vi "SaveModelFile.vi"(8 "error in":errorcluster, 11 "ItemNames":string[][](array[string])) -> (0 "error out":errorcluster)   [LabVIEW 2013]
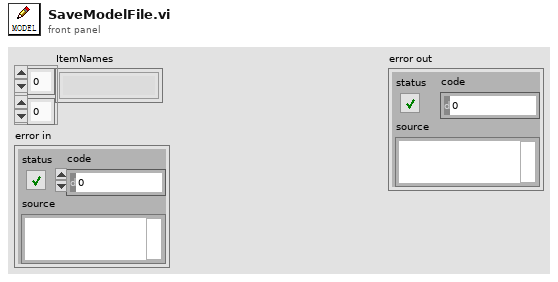
[diagram p1: front panel]
types:
  T1 = enum16{"open", "replace", "create", "open or create", "replace or create", "replace or create with confirmation"}
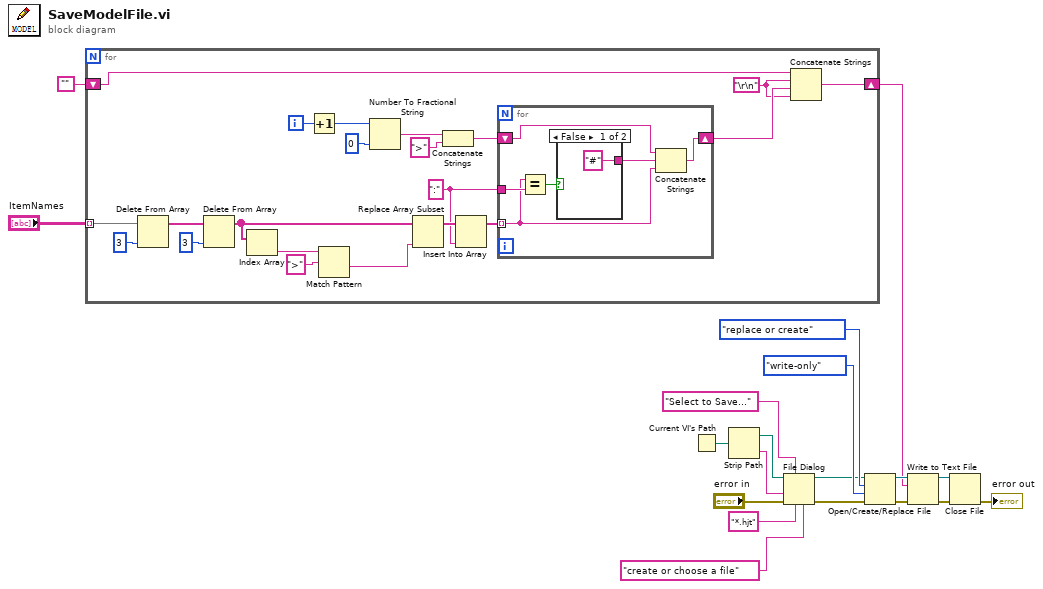
[diagram p0: block diagram]
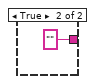
[diagram p2: hidden frame]
diagram:
  n1 = for {
    tunnel: "ItemNames" -> [w30] mode=indexing
    shift-right: [w34] -> w8
    shift-left: "" -> [w33]
    i -> [w40]
    w20 = ":" ("new element/subarray")
    w31 = "\r\n"
    n2 = Delete From Array(array=w30, index=3) -> (array with subset deleted=w27:string[])  [unwired: 1 in, 1 out]
    n3 = Delete From Array(array=w27, index=3) -> (array with subset deleted=w25:string[])  [unwired: 1 in, 1 out]
    n4 = Index Array(array=w25) -> (element=w26:string)  [unwired: 1 in]
    n5 = Increment(x=w40) -> (x+1=w39:i32)
    n6 = Match Pattern(string=w26, regular expression=">") -> (after substring=w24:string)  [unwired: 1 in, 3 out]
    n7 = Number To Fractional String(number=w39, precision (6)=i16 0) -> (F-format string=w38:string)  [unwired: 2 in]
    n8 = Replace Array Subset(array=w25, new element=w24) -> (w22:string[])  [unwired: 1 in]
    n9 = Concatenate Strings(w38, ">") -> (w36:string)
    n10 = Insert Into Array(array=w22, new element=w20) -> (w21:string[])  [unwired: 1 in]
    n11 = for {
      shift-right: [w45] -> w32
      shift-left: w36 -> [w46]
      tunnel: w21 -> [w43] mode=indexing
      tunnel: w20 -> [w44]
      n12 = Equal?(x=w43, y=w44) -> (x = y?=w42:bool)
      n13 = case shown="False" w42 {
        tunnel: ["#" ("string") ""] -> w41
        frame False {
        }
        frame True {
        }
      }
      n14 = Concatenate Strings(w46, w41, w43) -> (w45:string)
    }
    n15 = Concatenate Strings(w33, w31, w32, w31) -> (w34:string)
  }
  n16 = Current VI's Path() -> (path=w5:path)
  n17 = Strip Path(path=w5) -> (stripped path=w11:path, name=w12:string)
  n18 = File Dialog(4:"create or choose a file" ("pattern label"), 6:"*.hjt" ("pattern (all files)"), 7:"Select to Save..." ("prompt"), 8:"error in", 9:w12, 11:w11) -> (0:w14:errorcluster, 3:w13:path)  [unwired: 3 out]
  n19 = Open/Create/Replace File(file path (use dialog)=w13, error in=w14, operation (0:open)=T1."replace or create", access (0:read/write)=enum16{"read/write", "read-only", "write-only"}."write-only") -> (refnum out=w9:refnum<file>, error out=w10:errorcluster)  [unwired: 3 out]
  n20 = Write to Text File(file (use dialog)=w9, text=w8, error in=w10) -> (refnum out=w6:refnum<file>, error out=w7:errorcluster)  [unwired: 1 in, 1 out]
  n21 = Close File(refnum=w6, error in=w7) -> (error out=→"error out":errorcluster)  [unwired: 1 out]
